vi "SingleAcquisition.vi"() -> ()   [LabVIEW 2009]
uses:
  Data/GetPixelData16.vi
panel:
  in  "Centre AOI":bool
  in  "AOI Width":i64
  in  "AOI Height":i64
  in  "error status":errorcluster
  out "Pixel Encoding":string
  out "Intensity Graph":u16[][](graph)
  out "AOIStride":i64
  in  "PreAmp":string(combo)
  out "PixelData":u16[](array[numeric])
  out "ByteData":u8[](array[numeric])
  in  "ExposureTime":dbl
  out "ImageSizeBytes":i64
  out "Handle":i32
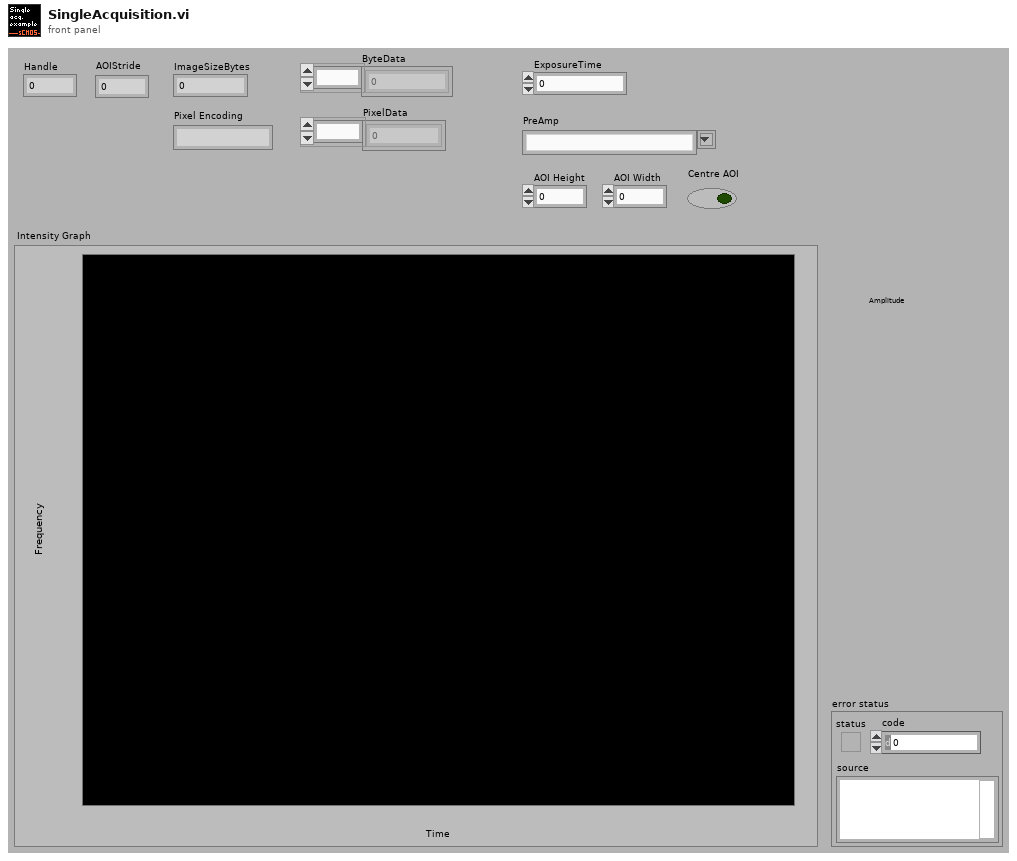
[diagram p1: front panel]
types:
  T1 = enum8{"Enabled", "Disabled", "Disabled and Grayed Out"}
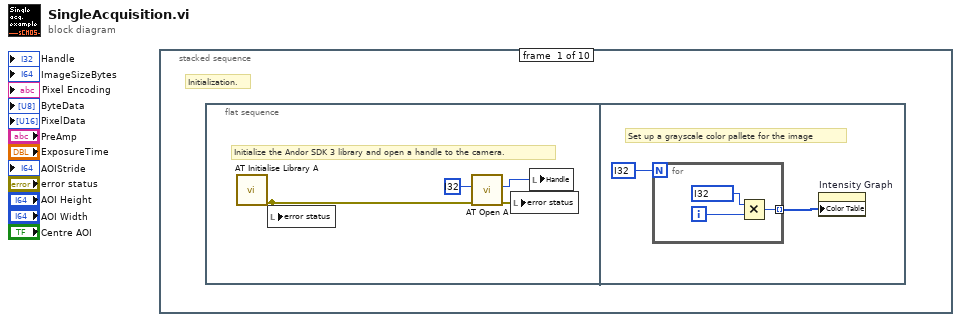
[diagram p0: block diagram]
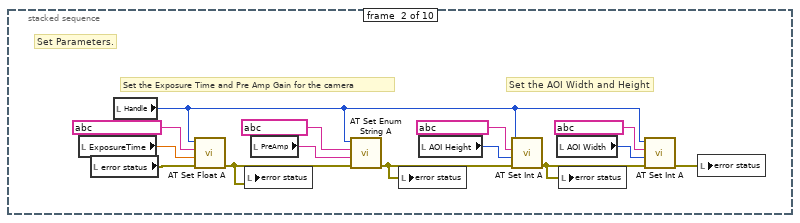
[diagram p2: hidden frame]
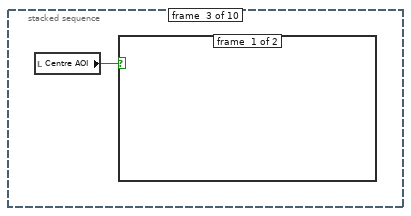
[diagram p3: hidden frame]
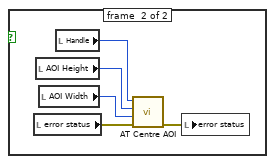
[diagram p4: hidden frame]
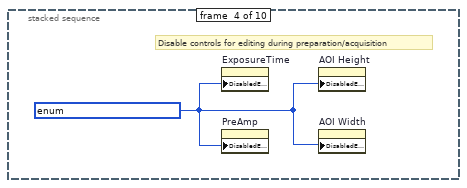
[diagram p5: hidden frame]
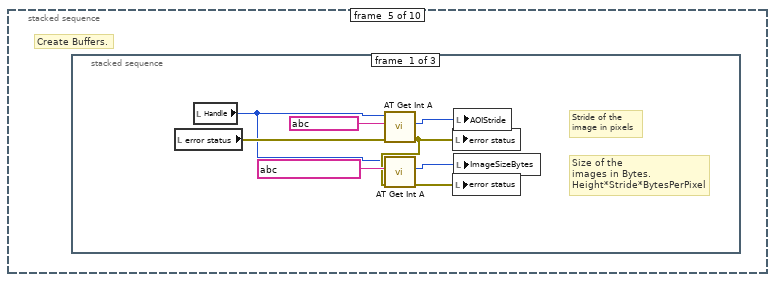
[diagram p6: hidden frame]
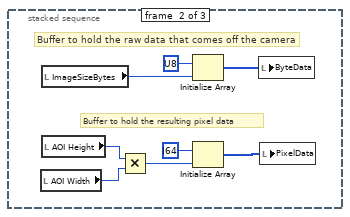
[diagram p7: hidden frame]
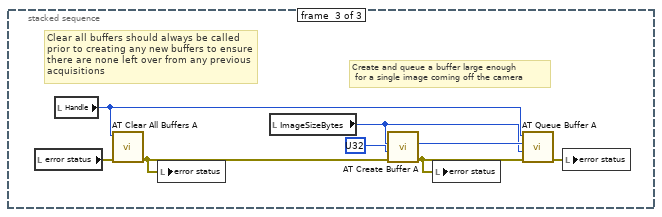
[diagram p8: hidden frame]
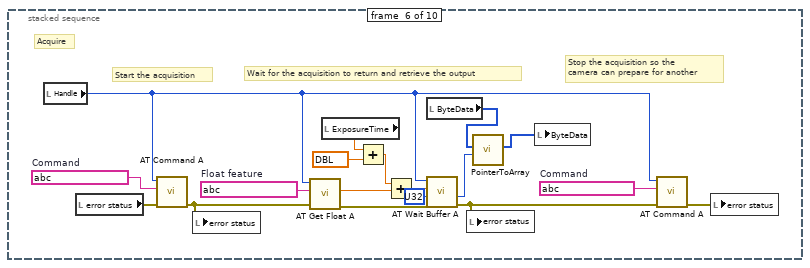
[diagram p9: hidden frame]
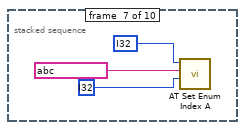
[diagram p10: hidden frame]
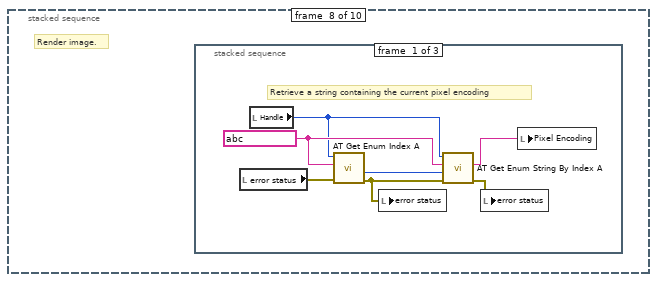
[diagram p11: hidden frame]
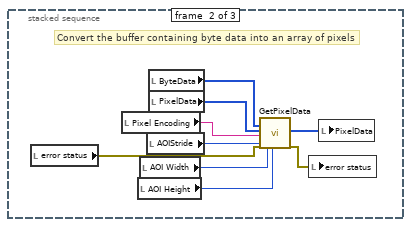
[diagram p12: hidden frame]
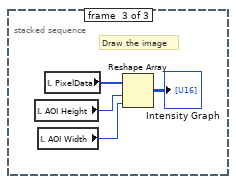
[diagram p13: hidden frame]
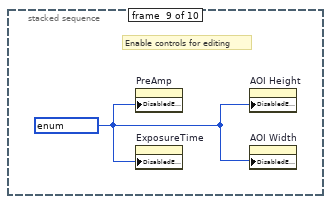
[diagram p14: hidden frame]
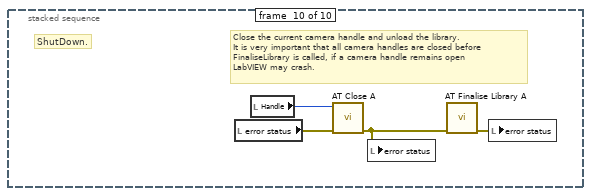
[diagram p15: hidden frame]
diagram:
  n1 = stacked-sequence {
    frame #0 {
      # "Initialization."
      n2 = flat-sequence {
        frame #0 {
          # "Initialize the Andor SDK 3 library and open a handle to the camera."
          n3 = call "AT Initialise Library A.vi"() -> ("error out"=w2:errorcluster)  [unwired: 10 in, 1 out]
          n4 = local write "error status"(w2) -> ()
          n5 = call "AT Open A.vi"("error in (no error)"=w2, "CameraIndex"=i32 ?) -> ("error out"=w1:errorcluster, "Handle"=w3:i32)  [unwired: 7 in, 1 out]
          n6 = local write "error status"(w1) -> ()
          n7 = local write "Handle"(w3) -> ()
        }
        frame #1 {
          # "Set up a grayscale color pallete for the image"
          n8 = for {
            N: i32 ? -> [_]
            tunnel: [w8] -> w5 mode=indexing
            i -> [w9]
            n9 = Multiply(x=i32 ?, y=w9) -> (x*y=w8:i32)
          }
          n10 = property on="Intensity Graph" class="IntGraph (strict)"("Color Table"=w5) -> ()  [unwired: 2 in, 2 out]
        }
      }
    }
    frame #1 {
      # "Set the AOI Width and Height"
      # "Set the Exposure Time and Pre Amp Gain for the camera"
      # "Set Parameters."
      n11 = local read "ExposureTime"() -> (w15:dbl)
      n12 = local read "error status"() -> (w19:errorcluster)
      n13 = local read "Handle"() -> (w10:i32)
      n14 = call "AT Set Float A.vi"("error in (no error)"=w19, "Value"=w15, "Feature"=string ? ("ExposureTime"), "Hndl"=w10) -> ("error out"=w22:errorcluster)  [unwired: 6 in, 1 out]
      n15 = local write "error status"(w22) -> ()
      n16 = local read "PreAmp"() -> (w23:string)
      n17 = call "AT Set Enum String A.vi"("error in (no error)"=w22, "String"=w23, "Feature"=string ? ("SimplePreAmpGainControl"), "Handle"=w10) -> ("error out"=w18:errorcluster)  [unwired: 6 in, 1 out]
      n18 = local write "error status"(w18) -> ()
      n19 = local read "AOI Height"() -> (w12:i64)
      n20 = call "AT Set Int A.vi"("error in (no error)"=w18, "Value"=w12, "Feature"=string ? ("Integer feature 2"), "Handle"=w10) -> ("error out"=w16:errorcluster)  [unwired: 6 in, 1 out]
      n21 = local read "AOI Width"() -> (w11:i64)
      n22 = local write "error status"(w16) -> ()
      n23 = call "AT Set Int A.vi"("error in (no error)"=w16, "Value"=w11, "Feature"=string ? ("Integer feature"), "Handle"=w10) -> ("error out"=w17:errorcluster)  [unwired: 6 in, 1 out]
      n24 = local write "error status"(w17) -> ()
    }
    frame #2 {
      n25 = local read "Centre AOI"() -> (w24:bool)
      n26 = case shown="True" w24 {
        frame #0 {
        }
        frame #1 {
          n27 = local read "error status"() -> (w29:errorcluster)
          n28 = local read "AOI Height"() -> (w26:i64)
          n29 = local read "AOI Width"() -> (w25:i64)
          n30 = local read "Handle"() -> (w27:i32)
          n31 = call "AT Centre AOI.vi"("error in (no error)"=w29, "AOI Width"=w25, "AOI Height"=w26, "Handle"=w27) -> ("error out"=w28:errorcluster)  [unwired: 7 in]
          n32 = local write "error status"(w28) -> ()
        }
      }
    }
    frame #3 {
      w30 = T1 ? ("Disabled")
      # "Disable controls for editing during preparation/acquisition"
      n33 = property on="ExposureTime" class="DigNum (strict)"("DisabledEnum"=w30) -> ()  [unwired: 2 in, 2 out]
      n34 = property on="PreAmp" class="CmbBox"("DisabledEnum"=w30) -> ()  [unwired: 2 in, 2 out]
      n35 = property on="AOI Height" class="DigNum (strict)"("DisabledEnum"=w30) -> ()  [unwired: 2 in, 2 out]
      n36 = property on="AOI Width" class="DigNum (strict)"("DisabledEnum"=w30) -> ()  [unwired: 2 in, 2 out]
    }
    frame #4 {
      # "Create Buffers."
      n37 = stacked-sequence {
        frame #0 {
          # "Stride of the\nimage in pixels"
          # "Size of the\nimages in Bytes.\nHeight*Stride*BytesPerPixel"
          n38 = local read "error status"() -> (w33:errorcluster)
          n39 = local read "Handle"() -> (w31:i32)
          n40 = call "AT Get Int A.vi"("error in (no error)"=w33, "Feature"=string ? ("Integer feature"), "Handle"=w31) -> ("error out"=w34:errorcluster, "Value"=w38:i64)  [unwired: 6 in, 1 out]
          n41 = call "AT Get Int A.vi"("error in (no error)"=w34, "Feature"=string ? ("Integer feature"), "Handle"=w31) -> ("error out"=w32:errorcluster, "Value"=w37:i64)  [unwired: 6 in, 1 out]
          n42 = local write "error status"(w34) -> ()
          n43 = local write "error status"(w32) -> ()
          n44 = local write "AOIStride"(w38) -> ()
          n45 = local write "ImageSizeBytes"(w37) -> ()
        }
        frame #1 {
          # "Buffer to hold the resulting pixel data"
          # "Buffer to hold the raw data that comes off the camera"
          n46 = local read "AOI Width"() -> (w45:i64)
          n47 = local read "ImageSizeBytes"() -> (w40:i64)
          n48 = local read "AOI Height"() -> (w44:i64)
          n49 = Multiply(x=w44, y=w45) -> (x*y=w39:i64)
          n50 = Initialize Array(u8 ?, w40) -> (w42:u8[])
          n51 = Initialize Array(i64 ?, w39) -> (w43:i64[])
          n52 = local write "ByteData"(w42) -> ()
          n53 = local write "PixelData"(w43) -> ()
        }
        frame #2 {
          # "Clear all buffers should always be called \nprior to creating any new buffers to ensure\nthere are none left over from any previous \nacquisitions"
          # "Create and queue a buffer large enough\n for a single image coming off the camera"
          n54 = local read "error status"() -> (w51:errorcluster)
          n55 = local read "Handle"() -> (w47:i32)
          n56 = call "AT Clear All Buffers A.vi"("error in (no error)"=w51, "Handle"=w47) -> ("error out"=w50:errorcluster)  [unwired: 8 in, 1 out]
          n57 = local write "error status"(w50) -> ()
          n58 = local read "ImageSizeBytes"() -> (w49:i64)
          n59 = call "AT Create Buffer A.vi"("error in (no error)"=w50, "Buffer"=u32 ?, "Size"=w49) -> ("error out"=w53:errorcluster, "Buffer out"=w54:u64)  [unwired: 6 in, 1 out]
          n60 = local write "error status"(w53) -> ()
          n61 = call "AT Queue Buffer A.vi"("error in (no error)"=w53, "PtrSize"=w49, "Ptr"=w54, "Handle"=w47) -> ("error out"=w52:errorcluster)  [unwired: 6 in, 1 out]
          n62 = local write "error status"(w52) -> ()
        }
      }
    }
    frame #5 {
      w63 = string ?  # Float feature
      w66 = string ?  # Command
      w71 = string ?  # Command
      # "Stop the acquisition so the \ncamera can prepare for another"
      # "Wait for the acquisition to return and retrieve the output"
      # "Start the acquisition"
      # "Acquire"
      n63 = local read "Handle"() -> (w70:i32)
      n64 = local read "error status"() -> (w72:errorcluster)
      n65 = call "AT Command A.vi"("error in (no error)"=w72, "Feature"=w71, "Handle"=w70) -> ("error out"=w69:errorcluster)  [unwired: 7 in, 1 out]
      n66 = local write "error status"(w69) -> ()
      n67 = call "AT Get Float A.vi"("error in (no error)"=w69, "Feature"=w63, "Handle"=w70) -> ("error out"=w68:errorcluster, "Value"=w64:dbl)  [unwired: 6 in, 1 out]
      n68 = local read "ExposureTime"() -> (w62:dbl)
      n69 = Add(x=w62, y=dbl ?) -> (x+y=w60:dbl)
      n70 = Add(x=w60, y=w64) -> (x+y=w65:dbl)
      n71 = local read "ByteData"() -> (w56:u8[])
      n72 = call "AT Wait Buffer A.vi"("error in (no error)"=w68, "Input buffer"=u32 ?, "Timeout"=w65, "Handle"=w70) -> ("error out"=w58:errorcluster, "Output buffer"=w55:u64)  [unwired: 4 in, 2 out]
      n73 = local write "error status"(w58) -> ()
      n74 = call "PointerToArray.vi"("Pointer In"=w55, "Array in"=w56) -> ("Array out"=w57:u8[])  [unwired: 8 in, 1 out]
      n75 = local write "ByteData"(w57) -> ()
      n76 = call "AT Command A.vi"("error in (no error)"=w58, "Feature"=w66, "Handle"=w70) -> ("error out"=w67:errorcluster)  [unwired: 7 in, 1 out]
      n77 = local write "error status"(w67) -> ()
    }
    frame #6 {
      n78 = call "AT Set Enum Index A.vi"("Value"=i32 ?, "Feature"=string ?, "Handle"=i32 ?) -> ()  [unwired: 7 in, 2 out]
    }
    frame #7 {
      # "Render image."
      n79 = stacked-sequence {
        frame #0 {
          w82 = string ?
          # "Retrieve a string containing the current pixel encoding"
          n80 = local read "error status"() -> (w78:errorcluster)
          n81 = local read "Handle"() -> (w80:i32)
          n82 = call "AT Get Enum Index A.vi"("error in (no error)"=w78, "Feature"=w82, "Handle"=w80) -> ("error out"=w79:errorcluster, "Value"=w81:i32)  [unwired: 6 in, 1 out]
          n83 = local write "error status"(w79) -> ()
          n84 = call "AT Get Enum String By Index A.vi"("error in (no error)"=w79, "Index"=w81, "Feature"=w82, "Handle"=w80) -> ("error out"=w77:errorcluster, "String"=w76:string)  [unwired: 5 in, 1 out]
          n85 = local write "error status"(w77) -> ()
          n86 = local write "Pixel Encoding"(w76) -> ()
        }
        frame #1 {
          # "Convert the buffer containing byte data into an array of pixels"
          n87 = local read "error status"() -> (w84:errorcluster)
          n88 = local read "Pixel Encoding"() -> (w83:string)
          n89 = local read "AOI Height"() -> (w89:i64)
          n90 = local read "AOI Width"() -> (w90:i64)
          n91 = local read "AOIStride"() -> (w88:i64)
          n92 = local read "ByteData"() -> (w86:u8[])
          n93 = local read "PixelData"() -> (w87:u16[])
          n94 = call-poly "GetPixelData.vi"("Input buffer"=w86, "Output buffer in"=w87, "Pixel Encoding"=w83, "Stride"=w88, "error in (no error)"=w84, "Width"=w90, "Height"=w89) -> ("Output buffer out"=w91:u16[], "error out"=w85:errorcluster)  [unwired: 10 in, 1 out]
          n95 = local write "error status"(w85) -> ()
          n96 = local write "PixelData"(w91) -> ()
        }
        frame #2 {
          # "Draw the image"
          n97 = local read "AOI Height"() -> (w94:i64)
          n98 = local read "AOI Width"() -> (w93:i64)
          n99 = local read "PixelData"() -> (w95:u16[])
          n100 = Reshape Array(w95, w94, w93) -> (→"Intensity Graph":u16[][])
        }
      }
    }
    frame #8 {
      w96 = T1 ? ("Disabled")
      # "Enable controls for editing"
      n101 = property on="PreAmp" class="CmbBox"("DisabledEnum"=w96) -> ()  [unwired: 2 in, 2 out]
      n102 = property on="ExposureTime" class="DigNum (strict)"("DisabledEnum"=w96) -> ()  [unwired: 2 in, 2 out]
      n103 = property on="AOI Height" class="DigNum (strict)"("DisabledEnum"=w96) -> ()  [unwired: 2 in, 2 out]
      n104 = property on="AOI Width" class="DigNum (strict)"("DisabledEnum"=w96) -> ()  [unwired: 2 in, 2 out]
    }
    frame #9 {
      # "Close the current camera handle and unload the library.\nIt is very important that all camera handles are closed before\nFinaliseLibrary is called, if a camera handle remains open \nLabVIEW may crash."
      # "ShutDown."
      n105 = local read "error status"() -> (w99:errorcluster)
      n106 = local read "Handle"() -> (w100:i32)
      n107 = call "AT Close A.vi"("error in (no error)"=w99, "Handle"=w100) -> ("error out"=w98:errorcluster)  [unwired: 8 in, 1 out]
      n108 = local write "error status"(w98) -> ()
      n109 = call "AT Finalise Library A.vi"("error in (no error)"=w98) -> ("error out"=w97:errorcluster)  [unwired: 9 in, 1 out]
      n110 = local write "error status"(w97) -> ()
    }
  }
